vi "visualizer main.vi"(8 "error in (no error)":errorcluster, 11 "Item Ref in":T4 format="%.0x") -> (0 "error out":errorcluster, 3 "Item Ref out":T4 format="%.0x")   [LabVIEW 2016, in "FPGA Resource Manager.lvlib"]
uses:
  FPGA Resource Manager.lvlib
  <vilib>/NI Veristand/Custom Device API/Custom Device Item Ref.ctl
  resource info.ctl
  viz_type.ctl
  viz_show.ctl
  Filters/Filter Parent/Filter.lvclass
  viz_filter.ctl
  viz_state.ctl
  <vilib>/NI VeriStand/Custom Device Tools/Custom Device Utility Library/Custom Device Utility Library.lvlib
  <vilib>/NI VeriStand/Custom Device API/Custom Device API.lvlib
panel:
  out "column width":i32[](array[numeric])
  in  "Options":enum32{"", "Sort", "Filter"}(tab)
  in  "Sort By...":T1 items=["RIO device", "resource", "input type", "datatype", "reserver"]
  in  "Invert?":bool
  in  "Filter Match":string
  in  "Filter Type":T2
  in  "Show":T3
  in  "Display":i32(listbox)
  out "Filter":refnum<class "Filter.lvclass">
  out "selected values":bool[](array[boolean])
  in  "table":i32(listbox)
  out "resource entries":T5[](array[typedef]) {"FPGA CD Ref" format="%.0x"; "reserver" format="%.0x"}
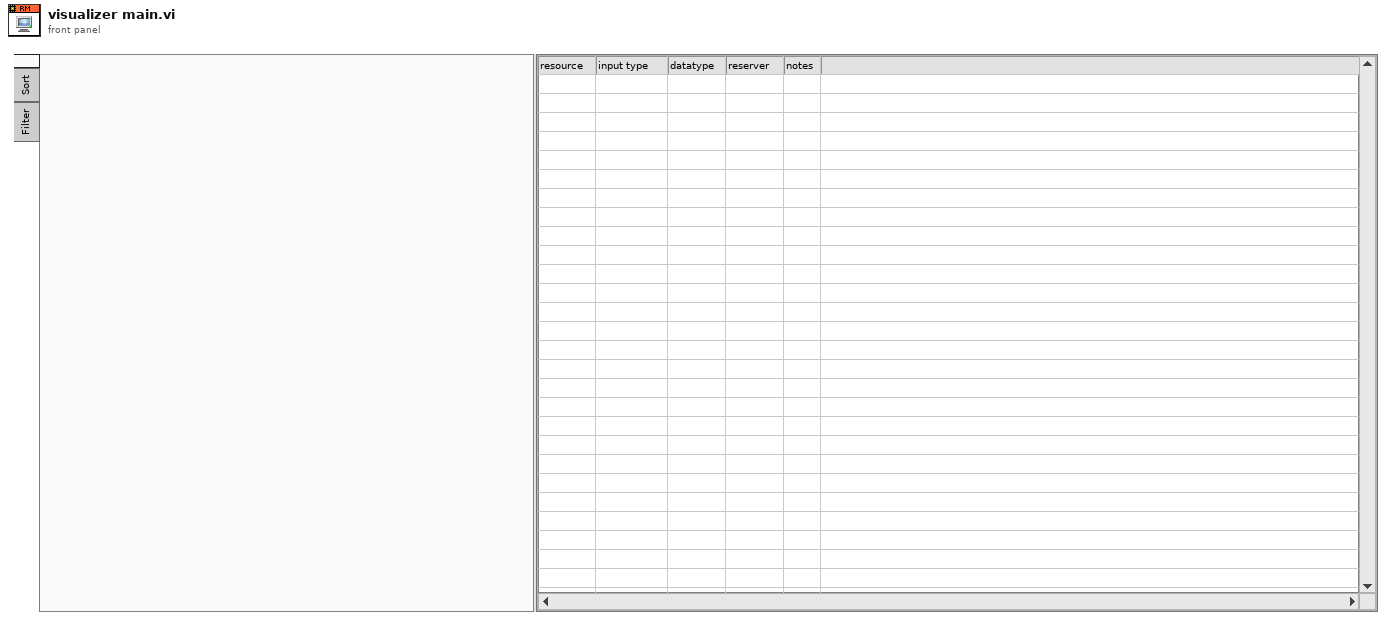
[diagram p1: front panel]
types:
  T1 = typedef "FPGA Resource Manager.lvlib/viz_type.ctl" = u16
  T2 = typedef "FPGA Resource Manager.lvlib/viz_filter.ctl" = enum16{"none", "RIO Device", "Resource Name", "Input Type", "Datatype"}
  T3 = typedef "FPGA Resource Manager.lvlib/viz_show.ctl" = enum16{"All", "Mapped", "Unmapped"}
  T4 = typedef "Custom Device API.lvlib/Custom Device Item Ref.ctl" = u64
  T5 = typedef "FPGA Resource Manager.lvlib/resource info.ctl" = cluster{"FPGA CD Ref":T4, "resource name":string, "input type":string, "datatype":string, "reserver":T4, "notes":string}
  T6 = typedef "FPGA Resource Manager.lvlib/viz_state.ctl" = enum16{"shutdown"}
  T7 = typedef "RM.Server.lvlib/viz_command.ctl" = cluster{"state":T8, "data":variant}
  T8 = typedef "RM.Server.lvlib/viz_state.ctl" = enum16{"shutdown"}
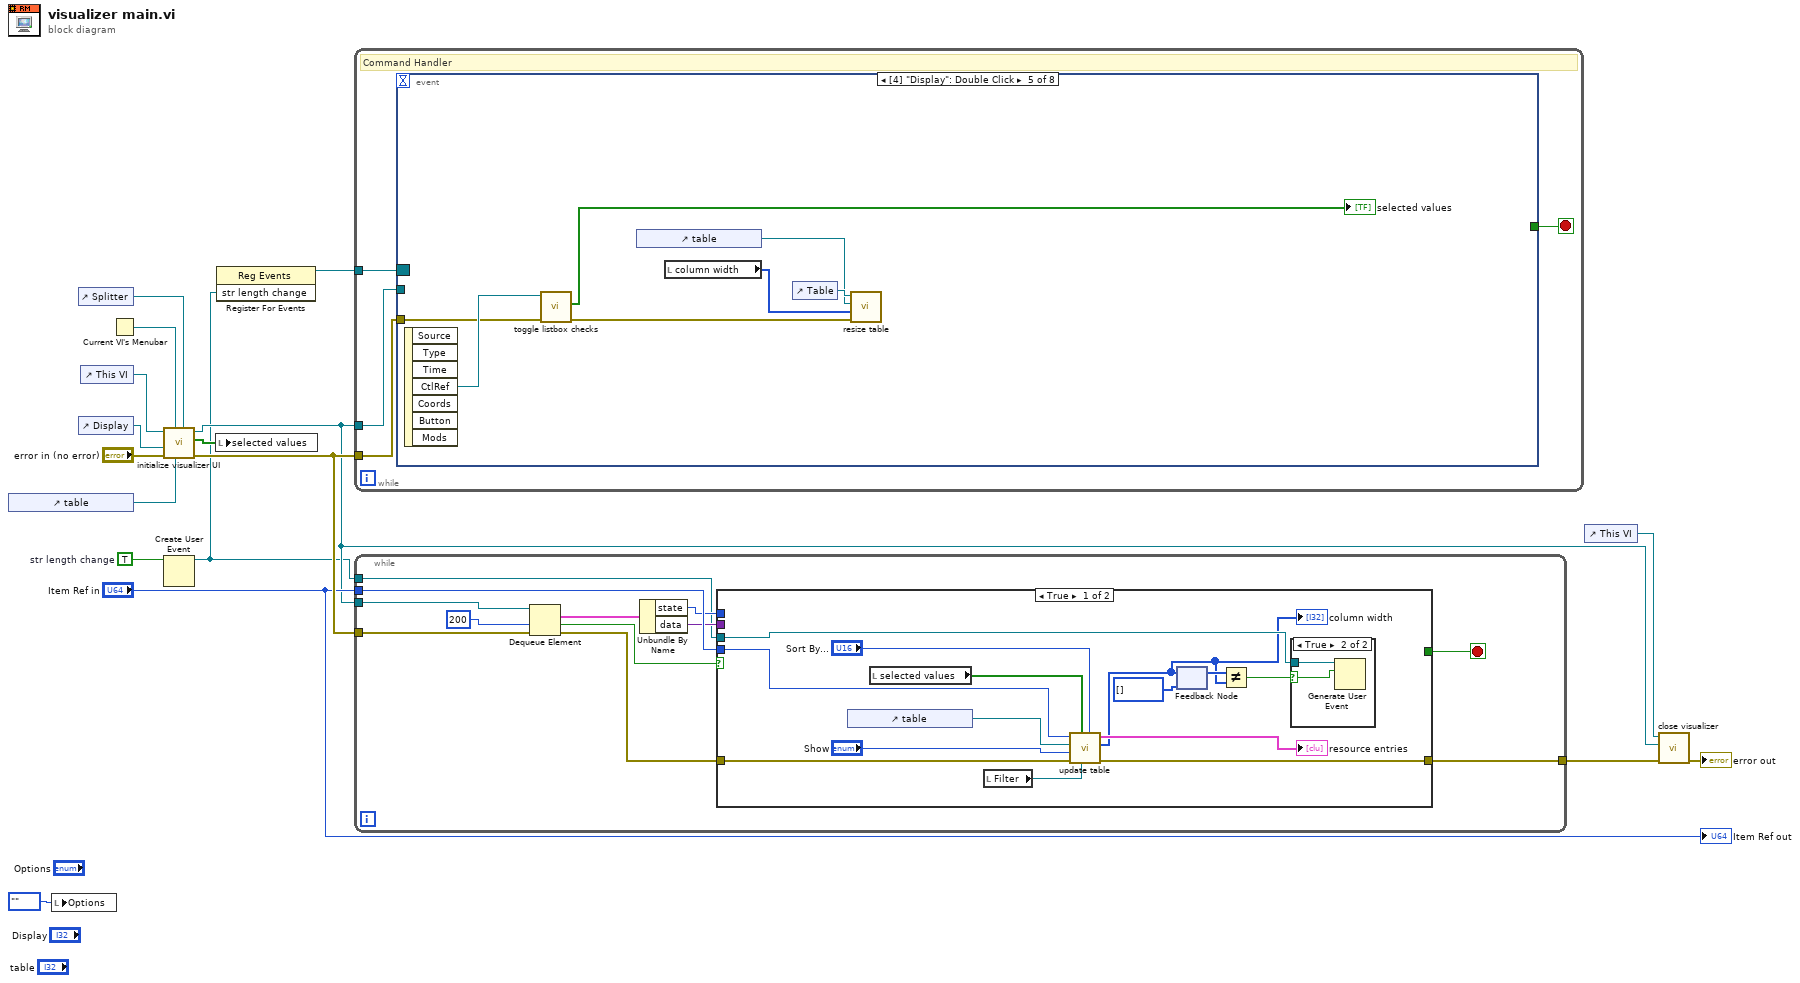
[diagram p0: block diagram]
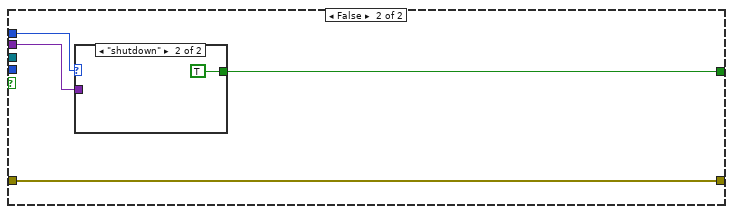
[diagram p3: hidden frame]
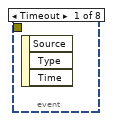
[diagram p5: hidden frame]
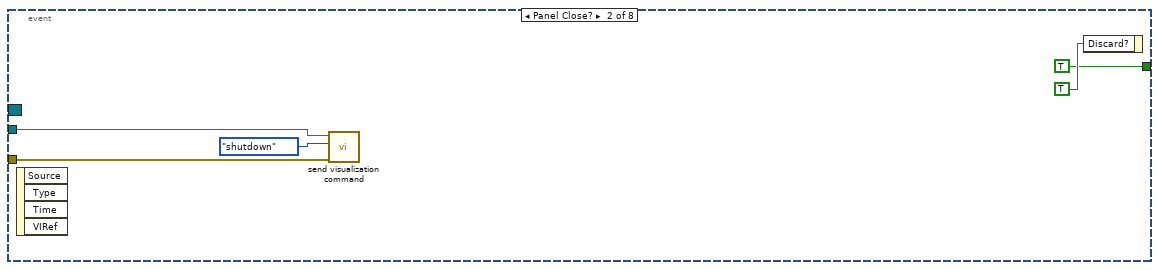
[diagram p6: hidden frame]
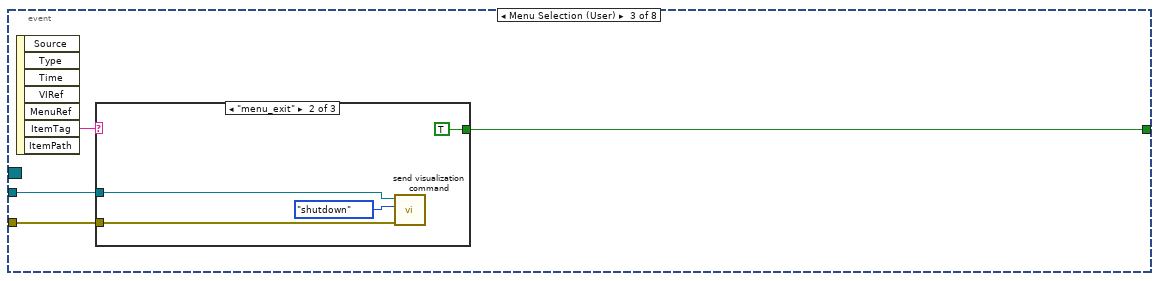
[diagram p7: hidden frame]
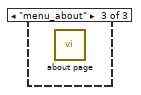
[diagram p9: hidden frame]
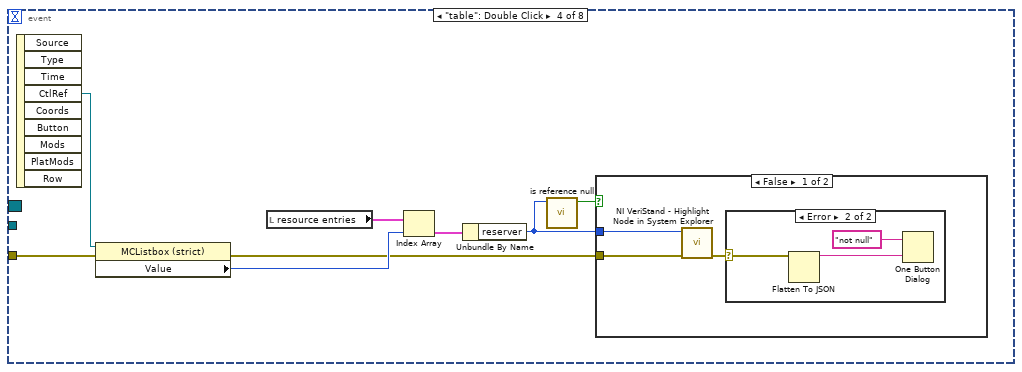
[diagram p10: hidden frame]
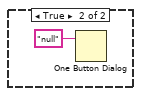
[diagram p12: hidden frame]
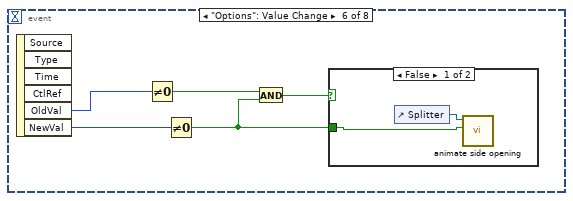
[diagram p13: hidden frame]
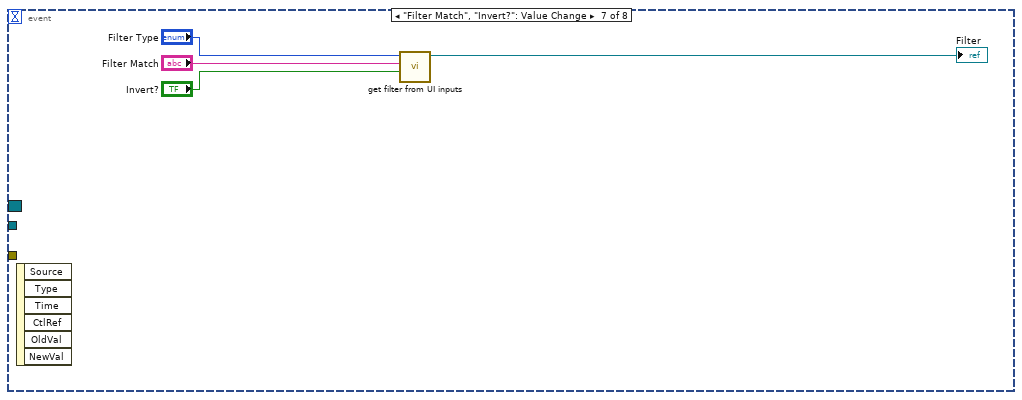
[diagram p15: hidden frame]
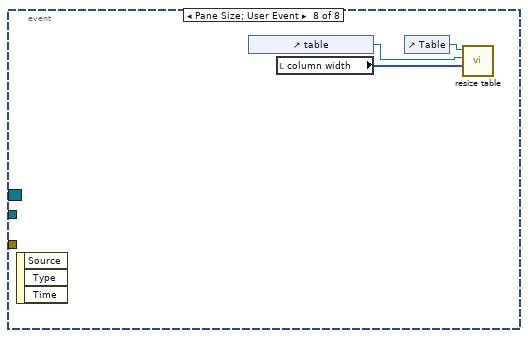
[diagram p16: hidden frame]
diagram:
  w3 = TRUE  # str length change
  n1 = control-ref of="table"() -> (w7:refnum<vi>)
  n2 = local write "Options"(enum32{"", "Sort", "Filter"}."" ("Options")) -> ()
  n3 = control-ref of="Splitter"() -> (w8:refnum<vi>)
  n4 = control-ref of="Display"() -> (w5:refnum<vi>)
  n5 = control-ref of="This VI"() -> (w14:refnum<vi>)
  n6 = Current VI's Menubar() -> (w9:refnum<k9>)
  n7 = call "initialize visualizer UI.vi"("Splitter"=w8, "MCLB Reference"=w7, "menu reference in"=w9, "error in (no error)"="error in (no error)", "display"=w5, "VI in"=w14) -> ("error out"=w16:errorcluster, "selected values"=w6:bool[], "Queue out"=w10:refnum<queue>)  [unwired: 3 in]
  n8 = Create User Event(user event datatype=w3) -> (user event=w1:refnum<user-event>)  [unwired: 1 in, 1 out]
  n9 = local write "selected values"(w6) -> ()
  n10 = register-events(w1) -> (reference out=w2:refnum<event-registration>)  [unwired: 2 in, 1 out]
  n11 = while {
    tunnel: w10 -> [w20]
    tunnel: w16 -> [w19]
    tunnel: w2 -> [w18]
    stop <- w21 stop-if-true
    # "Command Handler"
    n12 = event shown="[4] \"Display\": Double Click" {
      selector: w18 -> [_ _ _ _ _ _ _ _]
      dyn-events: _ -> [_ _ _ _ _ _ _ _]
      timeout: _ -> [_ _ _ _ _ _ _ _]
      tunnel: [_ TRUE w29 _ _ _ _ _] -> w21
      tunnel: w20 -> [_ w22 w28 _ _ _ _ _]
      tunnel: w19 -> [_ w23 w27 w41 w55 _ _ _]
      event Timeout {
        n13 = event-data() -> ()  [unwired: 1 in, 3 out]
      }
      event Panel Close? {
        n14 = event-data() -> ()  [unwired: 1 in, 4 out]
        n15 = call "send visualization command.vi"("error in (no error)"=w23, "state"=viz_state."shutdown" ("viz_state"), "Queue in"=w22) -> ()  [unwired: 8 in, 1 out]
        n16 = event-data("Discard?"=TRUE ("SilentShutdown")) -> ()  [unwired: 1 in, 1 out]
      }
      event Menu Selection (User) {
        n17 = event-data() -> ("ItemTag"=w30:string)  [unwired: 1 in, 6 out]
        n18 = case shown="\"menu_exit\"" w30 {
          tunnel: [_ TRUE _] -> w29
          tunnel: w28 -> [_ w33 _]
          tunnel: w27 -> [_ w31 _]
          frame Default {
          }
          frame "menu_exit" {
            n19 = call "send visualization command.vi"("error in (no error)"=w31, "state"=viz_state."shutdown" ("viz_state"), "Queue in"=w33) -> ()  [unwired: 8 in, 1 out]
          }
          frame "menu_about" {
            n20 = call "about page.vi"() -> ()  [unwired: 12 in]
          }
        }
      }
      event "table": Double Click {
        n21 = event-data() -> ("CtlRef"=w42:refnum<vi>)  [unwired: 1 in, 8 out]
        n22 = property class="MCListbox (strict)"(reference=w42, error in=w41) -> (error out=w39:errorcluster, "Value"=w40:i32)  [unwired: 1 out]
        n23 = local read "resource entries"() -> (w38:T5[])
        n24 = Index Array(array=w38, index=w40) -> (element=w37:T5)
        n25 = Unbundle By Name(w37) -> ("reserver"=w36:T4)
        n26 = call "is reference null.vi"("reserver"=w36) -> ("Boolean"=w35:bool)  [unwired: 10 in]
        n27 = case shown="False" w35 {
          tunnel: w39 -> [w45 _]
          tunnel: w36 -> [w44 _]
          frame False {
            n28 = call <vilib>:"NI VeriStand - Highlight Node in System Explorer.vi"("error in (no error)"=w45, "Item Ref in"=w44) -> ("error out"=w43:errorcluster)  [unwired: 8 in, 1 out]
            n29 = case shown="Error" w43 {
              selector: w43 -> [_ w47]
              frame No Error {
              }
              frame Error {
                n30 = Flatten To JSON(anything=w47) -> (JSON string=w46:string)  [unwired: 2 in, 1 out]
                n31 = One Button Dialog(message="not null", button name ("OK")=w46) -> ()  [unwired: 1 out]
              }
            }
          }
          frame True {
            n32 = One Button Dialog(message="null") -> ()  [unwired: 1 in, 1 out]
          }
        }
      }
      event "Display": Double Click {
        n33 = event-data() -> ("CtlRef"=w56:refnum<vi>)  [unwired: 1 in, 6 out]
        n34 = call "toggle listbox checks.vi"("error in (no error)"=w55, "ListBox in"=w56) -> ("error out"=w51:errorcluster, "selected values"=→"selected values":bool[])  [unwired: 8 in]
        n35 = control-ref of="table"() -> (w53:refnum<vi>)
        n36 = local read "column width"() -> (w52:i32[])
        n37 = control-ref of="Table"() -> (w54:refnum<vi>)
        n38 = call "resize table.vi"("error in (no error)"=w51, "Column Weights"=w52, "table"=w53, "Pane in"=w54) -> ()  [unwired: 7 in, 1 out]
      }
      event "Options": Value Change {
        n39 = event-data() -> ("OldVal"=w60:enum32{"", "Sort", "Filter"}, "NewVal"=w61:enum32{"", "Sort", "Filter"})  [unwired: 1 in, 4 out]
        n40 = Not Equal To 0?(x=w60) -> (x != 0?=w59:bool)
        n41 = Not Equal To 0?(x=w61) -> (x != 0?=w58:bool)
        n42 = And(x=w59, y=w58) -> (x .and. y?=w57:bool)
        n43 = case shown="False" w57 {
          tunnel: w58 -> [w62 _]
          frame False {
            n44 = control-ref of="Splitter"() -> (w63:refnum<vi>)
            n45 = call "animate side opening.vi"("expand/collapse"=w62, "Splitter in"=w63) -> ()  [unwired: 10 in]
          }
          frame True {
          }
        }
      }
      event "Filter Match", "Invert?": Value Change {
        n46 = event-data() -> ()  [unwired: 1 in, 6 out]
        n47 = call "get filter from UI inputs.vi"("NOT"="Invert?", "Filter Value"="Filter Match", "Filter Type"="Filter Type") -> ("Filter out"=→"Filter":refnum<class "Filter.lvclass">)  [unwired: 8 in]
      }
      event Pane Size; User Event {
        n48 = event-data() -> ()  [unwired: 1 in, 3 out]
        n49 = control-ref of="table"() -> (w69:refnum<vi>)
        n50 = local read "column width"() -> (w68:i32[])
        n51 = control-ref of="Table"() -> (w70:refnum<vi>)
        n52 = call "resize table.vi"("Column Weights"=w68, "table"=w69, "Pane in"=w70) -> ()  [unwired: 8 in, 1 out]
      }
    }
  }
  n53 = while {
    tunnel: w10 -> [w82]
    tunnel: w16 -> [w79]
    tunnel: "Item Ref in" -> [w77]
    tunnel: [w76] -> w13
    tunnel: w1 -> [w71]
    stop <- w80 stop-if-true
    n54 = Dequeue Element(queue=w82, timeout in ms (-1)=200, error in (no error)=w79) -> (element=w81:T7, timed out?=w74:bool, error out=w78:errorcluster)  [unwired: 1 out]
    n55 = Unbundle By Name(w81) -> ("state"=w73:T8, "data"=w72:variant)
    n56 = case shown="True" w74 {
      tunnel: [_ w102] -> w80
      tunnel: w78 -> [w96 w101]
      tunnel: w77 -> [w93 _]
      tunnel: [w95 w101] -> w76
      tunnel: w73 -> [_ w100]
      tunnel: w72 -> [_ w99]
      tunnel: w71 -> [w86 _]
      frame True {
        n57 = control-ref of="table"() -> (w94:refnum<vi>)
        n58 = local read "selected values"() -> (w92:bool[])
        n59 = local read "Filter"() -> (w89:refnum<class "Filter.lvclass">)
        n60 = call "update table.vi"("Sort By..."="Sort By...", "Filter in"=w89, "selected values"=w92, "error in (no error)"=w96, "Show"="Show", "MulticolumnListbox in"=w94, "Item Ref in"=w93) -> ("error out"=w95:errorcluster, "max string length in columns"=w84:i32[], "resource entries"=→"resource entries":T5[])  [unwired: 2 in]
        "column width" <- w84
        n61 = feedback-in #1(w84) -> ()
        n62 = feedback #1(i32[] [] ("max string length in columns")) -> (w87:i32[])
        n63 = Not Equal?(x=w87, y=w84) -> (x != y?=w85:bool)
        n64 = case shown="True" w85 {
          selector: w85 -> [_ w97]
          tunnel: w86 -> [_ w98]
          frame False {
          }
          frame True {
            n65 = Generate User Event(user event=w98, event data cluster=w97) -> ()  [unwired: 2 in, 2 out]
          }
        }
      }
      frame False {
        n66 = case shown="\"shutdown\"" w100 {
          tunnel: [_ TRUE] -> w102
          tunnel: w99 -> [_ _]
          frame Default {
          }
          frame "shutdown" {
          }
        }
      }
    }
  }
  n67 = control-ref of="This VI"() -> (w11:refnum<vi>)
  n68 = call "close visualizer.vi"("error in (no error)"=w13, "Queue in"=w10, "reference"=w11) -> ("error out"=→"error out":errorcluster)  [unwired: 8 in]
  "Item Ref out" <- "Item Ref in"
